vi "DCA Compute Power-Attenuation.vi"(1 "Measurement Values":T1) -> (0 "Power-Attenuation":dbl)   [LabVIEW 2011]
uses:
  TypeDefs/DCA Measurement Values.ctl
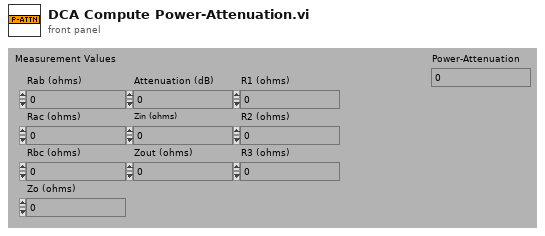
[diagram p1: front panel]
types:
  T1 = typedef "DCA Measurement Values.ctl" = cluster{"Rab (ohms)":dbl, "Rac (ohms)":dbl, "Rbc (ohms)":dbl, "Zo (ohms)":dbl, "Attenuation (dB)":dbl, "Zin (ohms)":dbl, "Zout (ohms)":dbl, "R1 (ohms)":dbl, "R2 (ohms)":dbl, "R3 (ohms)":dbl}
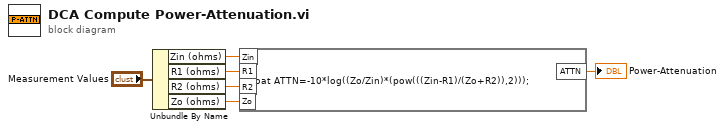
[diagram p0: block diagram]
diagram:
  n1 = Unbundle By Name("Measurement Values") -> ("Zin (ohms)"=w5:dbl, "R1 (ohms)"=w4:dbl, "R2 (ohms)"=w3:dbl, "Zo (ohms)"=w1:dbl)
  n2 = formula code="float ATTN=-10*log((Zo/Zin)*(pow(((Zin-R1)/(Zo+R2)),2)));"("Zin"=w5, "R1"=w4, "R2"=w3, "Zo"=w1) -> ("ATTN"=→"Power-Attenuation":dbl)
